vi "Create System Health Group.vi"(8 "error in (no error)":errorcluster, 11 "System Health Module in":refnum<class "System Health Module.lvclass">) -> (0 "error out":errorcluster, 3 "System Health Module out":refnum<class "System Health Module.lvclass">)   [LabVIEW 2020, in "Volatus.lvlib" / "System Health Module.lvclass"]
uses:
  System Health Module.lvclass
  System Health Module.lvclass/System Health Module.ctl
  Module/Module.lvclass
  VolatusConfig/Task/Task Config.lvclass
  C:/dev/lv20CE/relink/lv-volatus/Volatus/Module/Module.lvclass
  C:/dev/lv20CE/relink/lv-volatus/Volatus/System Health Module/System Health Module.lvclass
  lv-vecto/Vecto/Group DBL/Group DBL.lvclass
  C:/dev/lv20CE/relink/lv-vecto/Vecto/GroupAbstract/Group.lvclass
  C:/dev/lv20CE/relink/lv-vecto/Vecto/Group/Group DBL.lvclass
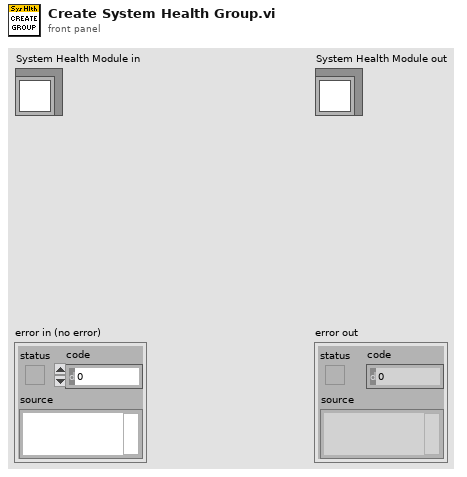
[diagram p1: front panel]
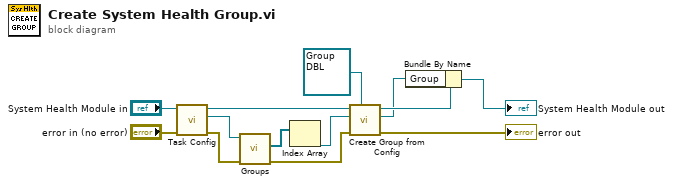
[diagram p0: block diagram]
diagram:
  n1 = call "Task Config.vi"("error in (no error)"="error in (no error)", "Module in"="System Health Module in") -> ("error out"=w9:errorcluster, "Task Config"=w13:refnum<class "Task Config.lvclass">, "Module out"=w8:refnum<class "System Health Module.lvclass">)  [unwired: 7 in]
  n2 = call "Groups.vi"("error in (no error)"=w9, "Task in"=w13) -> ("error out"=w6:errorcluster, "Groups"=w12:refnum<class "Group Config.lvclass">[])  [unwired: 7 in, 1 out]
  n3 = Index Array(array=w12) -> (element=w7:refnum<class "Group Config.lvclass">)  [unwired: 1 in]
  n4 = call "Create Group from Config.vi"("Group Type (Abstract)"=refnum<class "Group DBL.lvclass"> refnum ("Group"), "error in (no error)"=w6, "Group Config"=w7, "Module in"=w8) -> ("error out"=→"error out":errorcluster, "Group"=w2:refnum<class "Group DBL.lvclass">, "Module out"=w5:refnum<class "System Health Module.lvclass">)  [unwired: 5 in]
  n5 = Bundle By Name(cluster=w5, "Group"=w2) -> (→"System Health Module out":refnum<class "System Health Module.lvclass">)
